vi "Initialization SubVI.vi"(8 "error in (no error)":errorcluster, 11 "UI Data in":T1 {"Streak"."streak step" min=-1.0 max=1.0; "Streak"."streak length" min=-1.0 max=1.0}) -> (0 "error out":errorcluster, 3 "UI Data out":T1 {"Streak"."streak step" min=-1.0 max=1.0; "Streak"."streak length" min=-1.0 max=1.0})   [LabVIEW 2020]
uses:
  controls/UI Data.ctl
  controls/What animation enum.ctl
  controls/UI refnums.ctl
  controls/streak settings.ctl
  controls/timer control.ctl
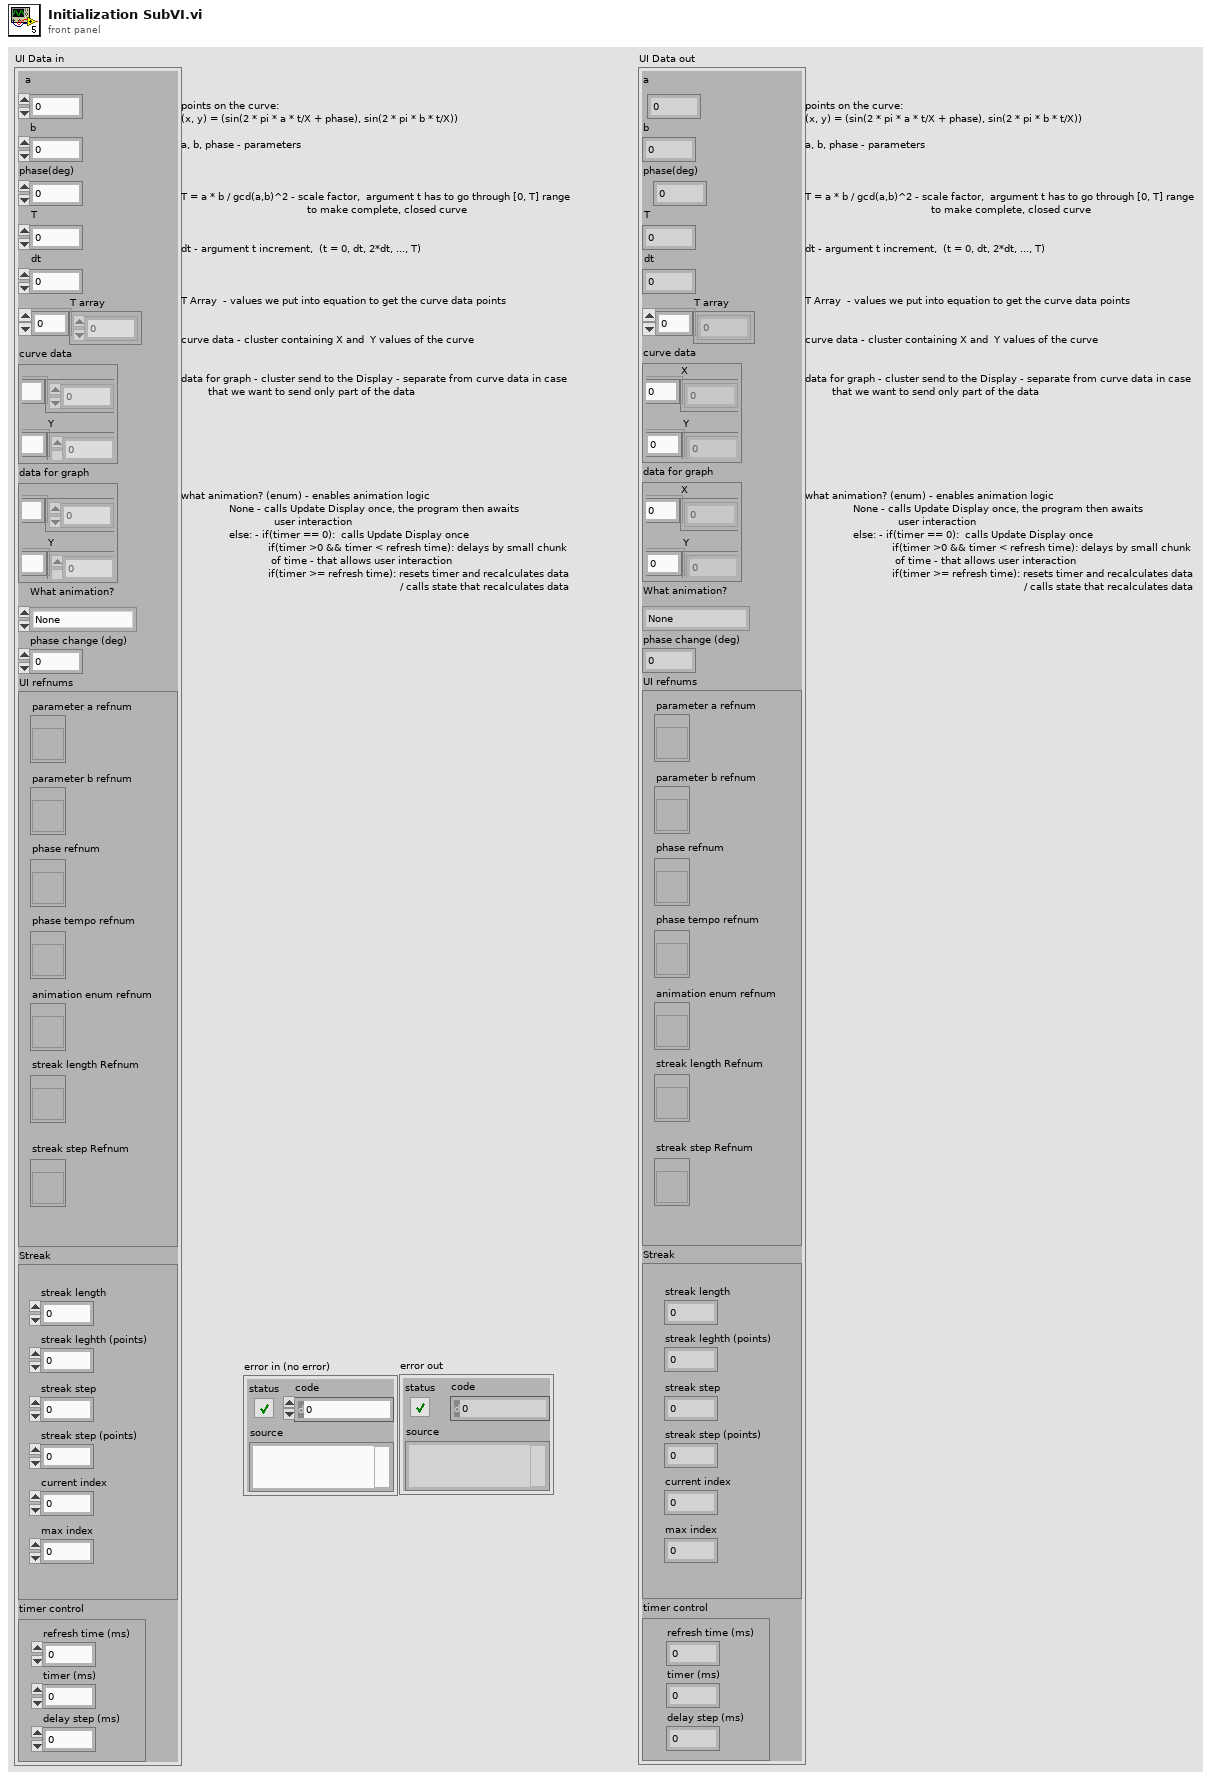
[diagram p1: front panel]
types:
  T1 = typedef "UI Data.ctl" = cluster{"a":i32, "b":i32, "phase(deg)":dbl, "T":i32, "dt":dbl, "T array":dbl[], "curve data":cluster{"X":dbl[], "Y ":dbl[]}, "data for graph":cluster{"X":dbl[], "Y ":dbl[]}, "What animation?":T2, "phase change (deg)":dbl, "UI refnums":T3, "Streak":T4, "timer control":T5}
  T2 = typedef "What animation enum.ctl" = enum16{"None", "Phase", "Streak"}
  T3 = typedef "UI refnums.ctl" = cluster{"parameter a refnum":refnum<vi>, "parameter b refnum":refnum<vi>, "phase refnum":refnum<vi>, "phase tempo refnum":refnum<vi>, "animation enum refnum":refnum<vi>, "streak length Refnum":refnum<vi>, "streak step Refnum":refnum<vi>}
  T4 = typedef "streak settings.ctl" = cluster{"streak length":dbl, "streak leghth (points)":i32, "streak step":dbl, "streak step (points)":i32, "current index":i32, "max index":i32}
  T5 = typedef "timer control.ctl" = cluster{"refresh time (ms)":dbl, "timer (ms)":dbl, "delay step (ms)":dbl}
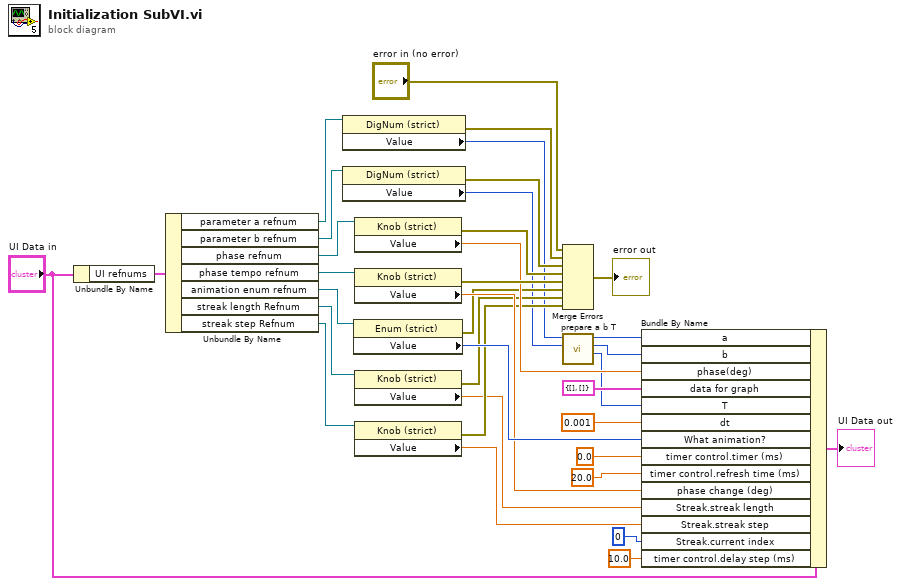
[diagram p0: block diagram]
diagram:
  n1 = Unbundle By Name("UI Data in") -> ("UI refnums"=w35:T3)
  n2 = Unbundle By Name(w35) -> ("parameter a refnum"=w30:refnum<vi>, "parameter b refnum"=w33:refnum<vi>, "phase refnum"=w32:refnum<vi>, "phase tempo refnum"=w31:refnum<vi>, "animation enum refnum"=w29:refnum<vi>, "streak length Refnum"=w11:refnum<vi>, "streak step Refnum"=w10:refnum<vi>)
  n3 = property class="DigNum (strict)"(reference=w30) -> (error out=w28:errorcluster, "Value"=w5:i32)  [unwired: 1 in, 1 out]
  n4 = property class="DigNum (strict)"(reference=w33) -> (error out=w27:errorcluster, "Value"=w4:i32)  [unwired: 1 in, 1 out]
  n5 = property class="Enum (strict)"(reference=w29) -> (error out=w13:errorcluster, "Value"=w23:T2)  [unwired: 1 in, 1 out]
  n6 = property class="Knob (strict)"(reference=w32) -> (error out=w26:errorcluster, "Value"=w17:dbl)  [unwired: 1 in, 1 out]
  n7 = property class="Knob (strict)"(reference=w31) -> (error out=w25:errorcluster, "Value"=w22:dbl)  [unwired: 1 in, 1 out]
  n8 = property class="Knob (strict)"(reference=w11) -> (error out=w9:errorcluster, "Value"=w7:dbl)  [unwired: 1 in, 1 out]
  n9 = property class="Knob (strict)"(reference=w10) -> (error out=w8:errorcluster, "Value"=w6:dbl)  [unwired: 1 in, 1 out]
  n10 = Merge Errors("error in (no error)", w28, w27, w26, w25, w13, w9, w8) -> (→"error out":errorcluster)
  n11 = call "prepare a b T.vi"("par b"=w4, "par a"=w5) -> ("T"=w1:i32, "b"=w2:i32, "a"=w3:i32)  [unwired: 7 in]
  n12 = Bundle By Name(cluster="UI Data in", "a"=w3, "b"=w2, "phase(deg)"=w17, "data for graph"=cluster{"X":dbl[], "Y ":dbl[]} {"X"=[], "Y "=[]}, "T"=w1, "dt"=0.001 ("dx"), "What animation?"=w23, "timer control.timer (ms)"=0.0 ("timer (ms)"), "timer control.refresh time (ms)"=20.0 ("refresh time (ms)"), "phase change (deg)"=w22, "Streak.streak length"=w7, "Streak.streak step"=w6, "Streak.current index"=0, "timer control.delay step (ms)"=10.0) -> (→"UI Data out":T1)
